vi "Initialize Instrument.vi"(8 "error in (no error)":errorcluster, 10 "Instr Resource Str":string, 11 "Simulated DMM.lvclass in":refnum<class "Simulated DMM.lvclass">) -> (0 "error out":errorcluster, 3 "Simulated DMM.lvclass out":refnum<class "Simulated DMM.lvclass">)   [LabVIEW 2010, in "Simulated DMM.lvclass"]
uses:
  Simulated DMM.lvclass
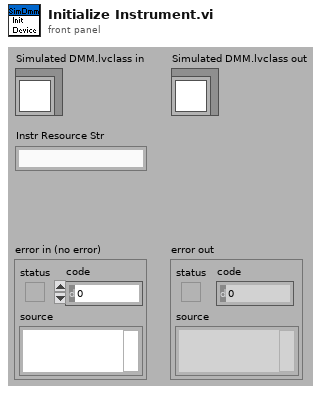
[diagram p1: front panel]
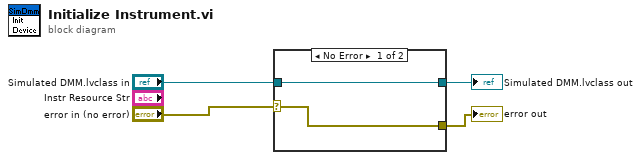
[diagram p0: block diagram]
diagram:
  n1 = case shown="No Error" "error in (no error)" {
    selector: "error in (no error)" -> [w5 w8]
    tunnel: [w5 w8] -> w3
    tunnel: "Simulated DMM.lvclass in" -> [w6 w7]
    tunnel: [w6 w7] -> w4
    frame No Error {
    }
    frame Error {
    }
  }
  "error out" <- w3
  "Simulated DMM.lvclass out" <- w4
